vi "UI Initialize.vi"(8 "error in (no error)":errorcluster, 11 "UI ActorTop in":refnum<class "UI_Up_Down.lvclass">) -> (0 "error out":errorcluster, 3 "UI ActorTop out":refnum<class "UI_Up_Down.lvclass">)   [LabVIEW 2021, in "UI_Up_Down.lvclass"]
doc: "UI: Initialize\n2015-03-18 16:27:22\n蒋松\njiangsong@outlook.com"
uses:
  UI_Up_Down.lvclass
  C:/Program Files (x86)/National Instruments/LabVIEW 2021/user.lib/John_Lib/AbstractActorTemplate/AbstractActorTemplate/UIActorTop.lvclass
  <userlib>/John_Lib/AbstractActorTemplate/AbstractActorTemplate/UIActorTop.lvclass
  <vilib>/ActorFramework/Actor/Actor.lvclass
  C:/Program Files (x86)/National Instruments/LabVIEW 2021/vi.lib/ActorFramework/Actor/Actor.lvclass
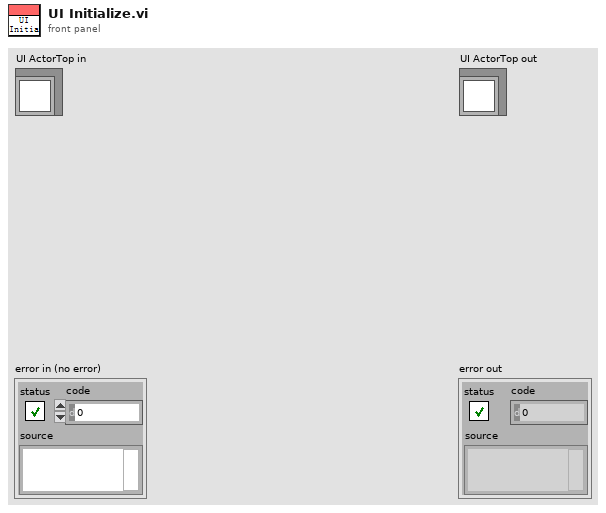
[diagram p1: front panel]
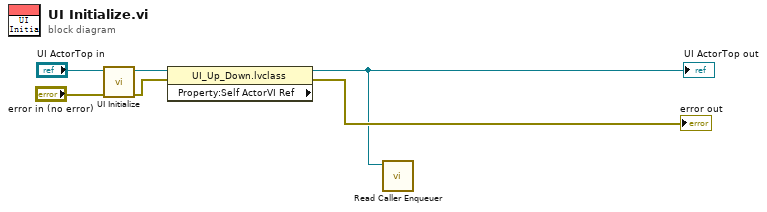
[diagram p0: block diagram]
diagram:
  n1 = call-parent "UI Initialize.vi"("error in (no error)"="error in (no error)", "UI ActorTop in"="UI ActorTop in") -> ("error out"=w3:errorcluster, "UI ActorTop out"=w5:refnum<class "UI_Up_Down.lvclass">)  [unwired: 8 in]
  n2 = property class="UI_Up_Down.lvclass" props=["Property:Self ActorVI Ref"](reference=w5, error in=w3) -> (reference out=w1:refnum<class "UI_Up_Down.lvclass">, error out=→"error out":errorcluster)  [unwired: 1 out]
  "UI ActorTop out" <- w1
  n3 = call <vilib>:"Read Caller Enqueuer.vi"("Actor"=w1) -> ()  [unwired: 10 in, 1 out]
